vi "Update_Best_Positions.vi"(0 "Target Value":dbl, 1 "Global Best Residual":dbl, 2 "Global Best Position":dbl, 5 "Particle Best Position":dbl[](array[numeric]), 7 "Particle Best Residual":dbl[](array[numeric]), 9 "Current Partical Value":dbl[](array[numeric]), 11 "Current Particle Position":dbl[](array[numeric])) -> (4 "Updated Best Particle Residual":dbl[](array[numeric]), 6 "Updated Particle Best Position":dbl[](array[numeric]), 8 "Current Partical Value Out":dbl[](array[numeric]), 10 "Current Particle Position Out":dbl[](array[numeric]), 13 "Updated Global Best Residual":dbl, 14 "Updated Global Best Position":dbl)   [LabVIEW 2011]
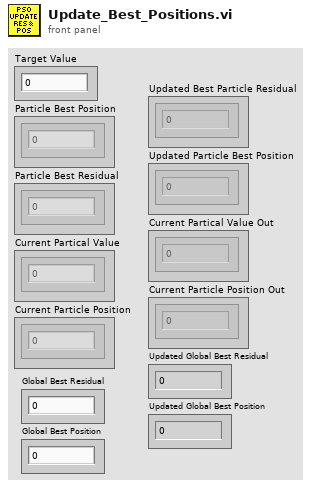
[diagram p1: front panel]
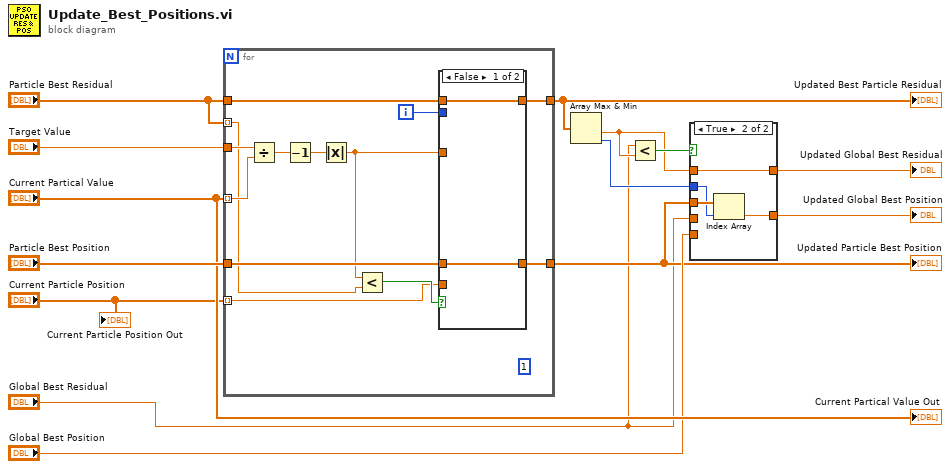
[diagram p0: block diagram]
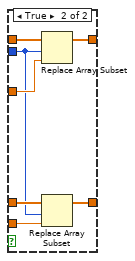
[diagram p3: hidden frame]
diagram:
  n1 = for {
    tunnel: "Particle Best Position" -> [w24]
    tunnel: "Target Value" -> [w22]
    tunnel: "Current Partical Value" -> [w23] mode=indexing
    tunnel: "Particle Best Residual" -> [w26]
    tunnel: "Current Particle Position" -> [w18] mode=indexing
    tunnel: [w17] -> w7
    tunnel: [w16] -> w10
    tunnel: "Particle Best Residual" -> [w15] mode=indexing
    i -> [w25]
    (unwired) 1 ("sample length")
    n2 = Divide(x=w22, y=w23) -> (x/y=w21:dbl)
    n3 = Decrement(x=w21) -> (x-1=w20:dbl)
    n4 = Absolute Value(x=w20) -> (abs(x)=w19:dbl)
    n5 = Less?(x=w19, y=w15) -> (x < y?=w27:bool)
    n6 = case shown="False" w27 {
      tunnel: w26 -> [w28 w36]
      tunnel: w19 -> [_ w35]
      tunnel: w25 -> [_ w33]
      tunnel: w24 -> [w29 w34]
      tunnel: w18 -> [_ w32]
      tunnel: [w29 w31] -> w17
      tunnel: [w28 w30] -> w16
      frame False {
      }
      frame True {
        n7 = Replace Array Subset(array=w36, new element=w35, index=w33) -> (w30:dbl[])
        n8 = Replace Array Subset(array=w34, new element=w32, index=w33) -> (w31:dbl[])
      }
    }
  }
  "Updated Best Particle Residual" <- w10
  "Updated Particle Best Position" <- w7
  n9 = Array Max & Min(array=w10) -> (min value=w5:dbl, min index (indices)=w6:i32)  [unwired: 2 out]
  n10 = Less?(x="Global Best Residual", y=w5) -> (x < y?=w9:bool)
  n11 = case shown="True" w9 {
    tunnel: "Global Best Position" -> [w38 _]
    tunnel: w7 -> [_ w42]
    tunnel: w6 -> [_ w41]
    tunnel: w5 -> [_ w39]
    tunnel: "Global Best Residual" -> [w37 _]
    tunnel: [w38 w40] -> w3
    tunnel: [w37 w39] -> w2
    frame False {
    }
    frame True {
      n12 = Index Array(array=w42, index=w41) -> (element=w40:dbl)
    }
  }
  "Updated Global Best Position" <- w3
  "Updated Global Best Residual" <- w2
  "Current Partical Value Out" <- "Current Partical Value"
  "Current Particle Position Out" <- "Current Particle Position"
